vi "resetAll.vi"(8 "error in (no error)":errorcluster, 11 "StaticOutputEditor in":refnum<class "StaticOutputEditor.lvclass">) -> (0 "error out":errorcluster, 3 "StaticOutputEditor out":refnum<class "StaticOutputEditor.lvclass">)   [LabVIEW 2011, in "Views.lvlib" / "ScriptEditor.lvlib" / "StaticOutputEditor.lvclass"]
uses:
  StaticOutputEditor.lvclass
  StaticOutputEditor.lvclass/StaticOutputEditor.ctl
  Hal/HWController/HWControllerEvents/HWControllerEvents.lvclass
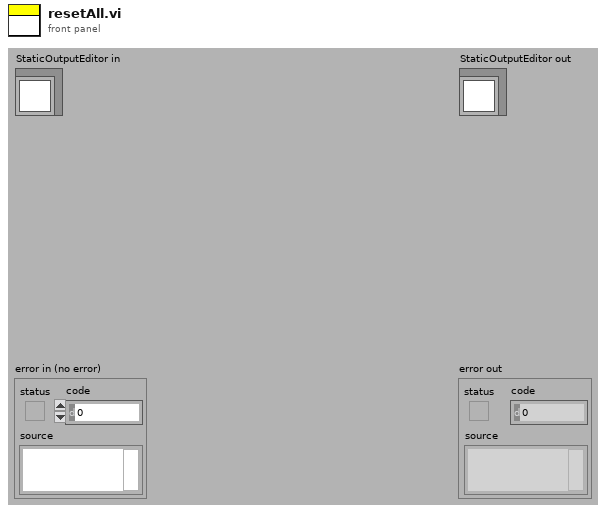
[diagram p1: front panel]
types:
  T1 = enum16{"start", "stop", "statusInquiry", "configure", "resetError", "resourcesInquiry", "reserveResources", "initialise", "resetAllChannels", "staticUpdate", "close", "HWStatus", "error", "resourcesAvailable", "resourcesReserved", "compilerError", "compiledScript", "compilingScript", "runScript", "configureCompiledScript"}
  T2 = cluster{"channelName":string, "value":string, "freq":string, "phase":string}[]
  T3 = cluster{"incomingEventTypes":cluster{"start":cluster{"Boolean":bool}, "stop":cluster{"Boolean":bool}, "statusInquiry":cluster{"Boolean":bool}, "configure":cluster{"DPScriptPath":path, "TimeStamp":string, "HWLoop?":bool}, "resetError":cluster{"Boolean":bool}, "resourcesInquiry":cluster{"Boolean":bool}, "reserveResources":cluster{"HWList":string[]}, "initialise":cluster{"HWList":string[]}, "close":cluster{"Boolean":bool}, "resetAllChannels":cluster{"Boolean":bool}, "staticChannelUpdate":cluster{"channel_address":string, "calibratedValue":dbl}, "runScript":cluster{"DPScriptPath":path, "TimeStamp":string, "HWLoop?":bool}, "compilingScript":cluster{"Path":path}, "compiledScript":cluster{"Path":path, "timeCompileAt":string}, "compilerError":cluster{"Path":path}, "configureCompiledScript":cluster{"DPScriptPath":path, "TimeStamp":string, "HWLoop?":bool, "CompiledScript":cluster{"ScriptListCompiler.lvclass":refnum<class "ScriptListCompiler.lvclass">, "aoChannels":refnum<class "AnalogOutput.lvclass">[], "doChannels":refnum<class "DigitalOutput.lvclass">[], "rfChannels":refnum<class "DDSOutput.lvclass">[]}}, "restartCompiler":cluster{"restart":bool}, "staticRfChannelUpdate":cluster{"channel_address":string, "Output":cluster{"Frequency(MHz)":dbl, "Amplitude":dbl, "Phase":dbl, "OutputForm":enum16{"Sine", "Square", "Triangle", "Arbitrary"}}}, "cameraUpdate":cluster{"Camera":string, "Type":string, "settings":path}}, "outgoingEventTypes":cluster{"HWStatus":cluster{"status":enum16{"Ready", "Compiling", "Configured", "Running", "Stopping", "Unresolved Error"}}, "error":cluster{"error out":errorcluster}, "resourcesAvailable":cluster{"availableHWList":string[], "reservedHWList":string[]}, "resourcesReserved":cluster{"reservedHWList":string[]}}}
  T4 = cluster{"channelName":string, "value":string, "freq":string, "phase":string}
  T5 = cluster{"eventId":enum16{"start", "stop", "statusInquiry", "configure", "resetError", "resourcesInquiry", "reserveResources", "initialise", "resetAllChannels", "staticUpdate", "close", "HWStatus", "error", "resourcesAvailable", "resourcesReserved", "compilerError", "compiledScript", "compilingScript", "runScript", "configureCompiledScript"}, "resetAllChannels":cluster{"Boolean":bool}}
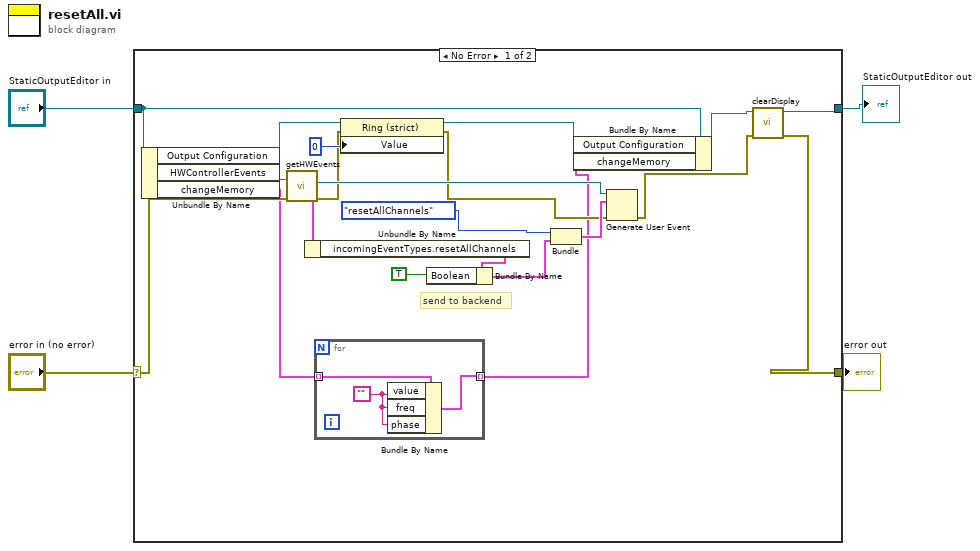
[diagram p0: block diagram]
diagram:
  n1 = case shown="No Error" "error in (no error)" {
    selector: "error in (no error)" -> [w20 w30]
    tunnel: [w5 w30] -> w3
    tunnel: [w8 w29] -> w1
    tunnel: "StaticOutputEditor in" -> [w12 w29]
    frame No Error {
      # "send to backend"
      n2 = Unbundle By Name(w12) -> ("Output Configuration"=w17:refnum<vi>, "HWControllerEvents"=w25:refnum<class "HWControllerEvents.lvclass">, "changeMemory"=w10:T2)
      n3 = call-dynamic "getHWEvents.vi"("error in (no error)"=w20, "HWControllerEvents in"=w25) -> ("error out"=w14:errorcluster, "eventDataTypes"=w18:T3, "HWCEvent"=w21:refnum<user-event>)  [unwired: 6 in, 1 out]
      n4 = Unbundle By Name(w18) -> ("incomingEventTypes.resetAllChannels"=w24:cluster{"Boolean":bool})
      n5 = for {
        tunnel: w10 -> [w28] mode=indexing
        tunnel: [w26] -> w9 mode=indexing
        w27 = ""
        n6 = Bundle By Name(cluster=w28, "value"=w27, "freq"=w27, "phase"=w27) -> (w26:T4)
      }
      n7 = property class="Ring (strict)"(reference=w17, error in=w14, "Value"=0) -> (reference out=w15:refnum<vi>, error out=w13:errorcluster)
      n8 = Bundle By Name(cluster=w24, "Boolean"=TRUE) -> (w23:cluster{"Boolean":bool})
      n9 = Bundle("eventId"=T1."resetAllChannels", "resetAllChannels"=w23) -> (w22:T5)  [unwired: 1 in]
      n10 = Bundle By Name(cluster=w12, "Output Configuration"=w15, "changeMemory"=w9) -> (w7:refnum<class "StaticOutputEditor.lvclass">)
      n11 = Generate User Event(user event=w21, event data cluster=w22, error in=w13) -> (error out=w6:errorcluster)  [unwired: 1 out]
      n12 = call "clearDisplay.vi"("error in (no error)"=w6, "StaticOutputEditor in"=w7) -> ("error out"=w5:errorcluster, "StaticOutputEditor out"=w8:refnum<class "StaticOutputEditor.lvclass">)  [unwired: 8 in]
    }
    frame Error {
    }
  }
  "error out" <- w3
  "StaticOutputEditor out" <- w1
